vi "Read Events.vi"(8 "error in (no error)":errorcluster, 11 "Recipe State Data in":refnum<class "Recipe State Data.lvclass">) -> (0 "error out":errorcluster, 2 "Events":T1, 3 "Recipe State Data out":refnum<class "Recipe State Data.lvclass">)   [LabVIEW 2022 SP3, in "Recipe State Data.lvclass"]
uses:
  Recipe State Data.lvclass
  Recipe State Data.lvclass/Recipe State Data.ctl
  Events.ctl
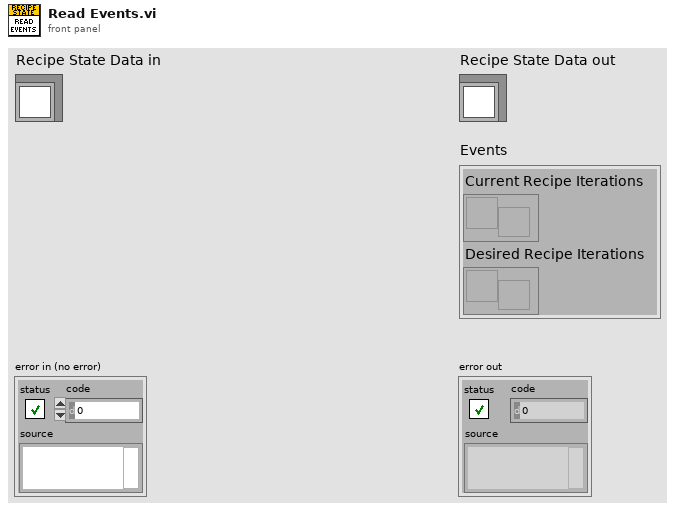
[diagram p1: front panel]
types:
  T1 = typedef "Recipe State Data.lvclass/Events.ctl" = cluster{"Current Recipe Iterations":refnum<user-event>, "Desired Recipe Iterations":refnum<user-event>}
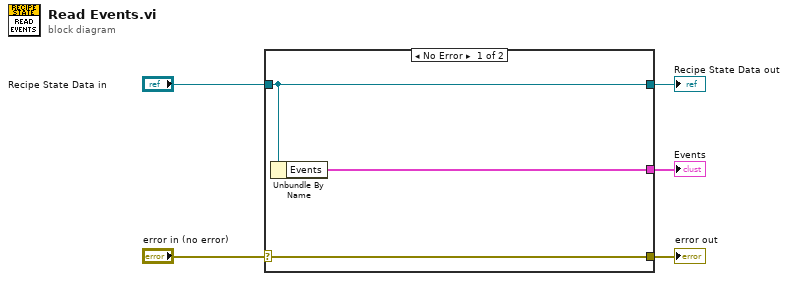
[diagram p0: block diagram]
diagram:
  n1 = case shown="No Error" "error in (no error)" {
    selector: "error in (no error)" -> [w8 w9]
    tunnel: [w8 w9] -> w4
    tunnel: [w7 w10] -> w2
    tunnel: "Recipe State Data in" -> [w7 w10]
    tunnel: [w6 _] -> w1
    frame No Error {
      n2 = Unbundle By Name(w7) -> ("Events"=w6:T1)
    }
    frame Error {
    }
  }
  "error out" <- w4
  "Recipe State Data out" <- w2
  "Events" <- w1
